vi "pyCode getAllData.vi"(8 "error in (no error)":errorcluster, 11 "pyCode in":refnum<class "pyCode.lvclass">) -> (0 "error out":errorcluster, 2 "response":string, 3 "pyCode out":refnum<class "pyCode.lvclass">)   [LabVIEW 2018, in "pyCode.lvclass"]
uses:
  pyCode.lvclass
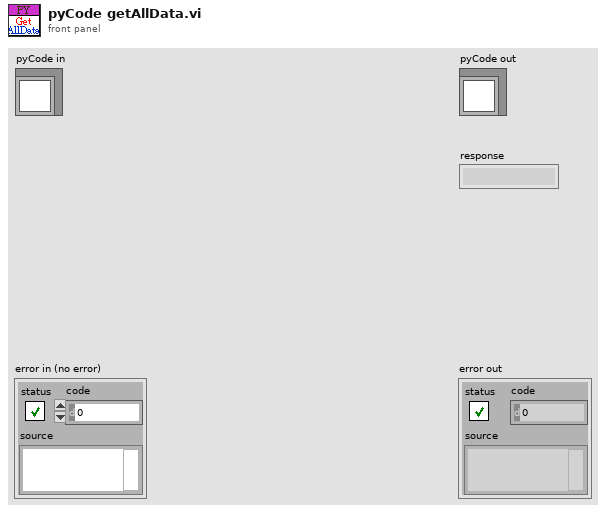
[diagram p1: front panel]
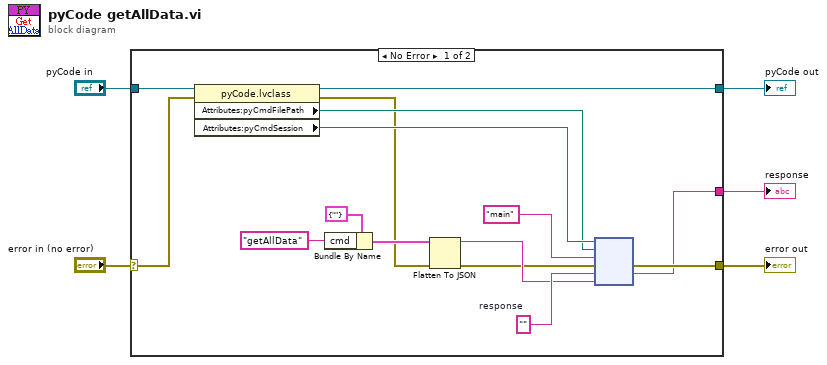
[diagram p0: block diagram]
diagram:
  n1 = case shown="No Error" "error in (no error)" {
    selector: "error in (no error)" -> [w10 w22]
    tunnel: [w8 w22] -> w3
    tunnel: [w19 w21] -> w4
    tunnel: "pyCode in" -> [w20 w21]
    tunnel: [w6 _] -> w1
    frame No Error {
      w15 = ""  # response
      n2 = property class="pyCode.lvclass"(reference=w20, error in=w10) -> (reference out=w19:refnum<class "pyCode.lvclass">, error out=w9:errorcluster, "Attributes:pyCmdFilePath"=w17:path, "Attributes:pyCmdSession"=w18:refnum<k35>)
      n3 = Bundle By Name(cluster=cluster{"cmd":string} {"cmd"=""}, "cmd"="getAllData") -> (w13:cluster{"cmd":string})
      n4 = Flatten To JSON(anything=w13, error in (no error)=w9) -> (JSON string=w12:string, 11:w11:errorcluster)  [unwired: 1 in]
      n5 = node(w18, w17, "main" ("function name"), w11, w15, w12) -> (w8:errorcluster, w6:string)  [unwired: 1 in, 3 out]
    }
    frame Error {
    }
  }
  "error out" <- w3
  "pyCode out" <- w4
  "response" <- w1
